vi "MIMIC RecvCommand.vi"(4 "error in":errorcluster, 7 "VISA resource name":refnum<visa-resource-name>) -> (0 "error out":errorcluster, 1 "Receive_buffer":u8[](array[numeric]), 2 "Receive Buffer_MP":u8[](array[numeric]), 3 "VISA resource name OUT":refnum<visa-resource-name>)   [LabVIEW 2014]
panel:
  out "IndexArray":u8[](array[numeric])
  out "Numeric":dbl
  out "Write Time":u32
  out "Read Time":u32
  out "return count":u32
  out "NUM_BYTES":u32
  out "Index":u32
  out "continue_flag":bool=TRUE
  out "STRT_TIME":u32
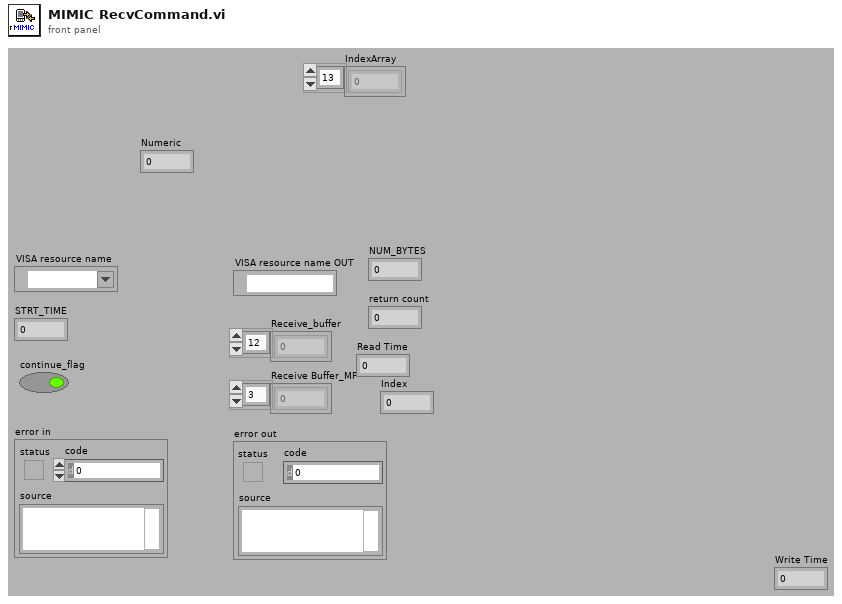
[diagram p1: front panel]
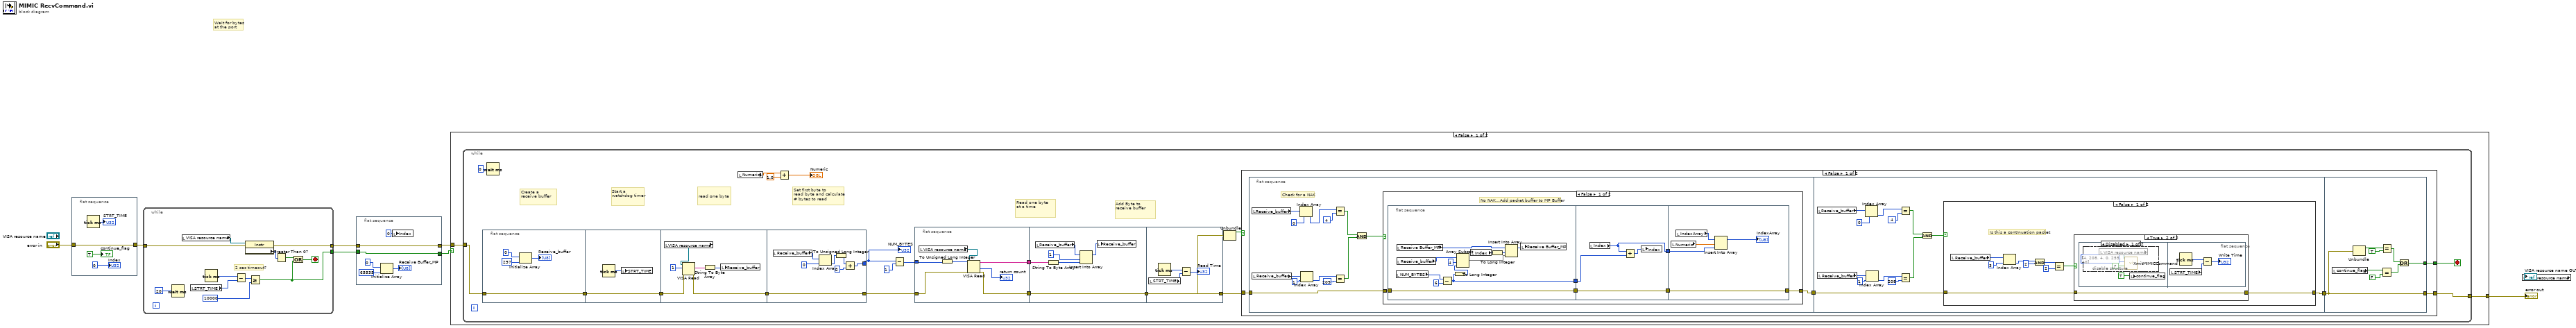
[diagram p0: block diagram]
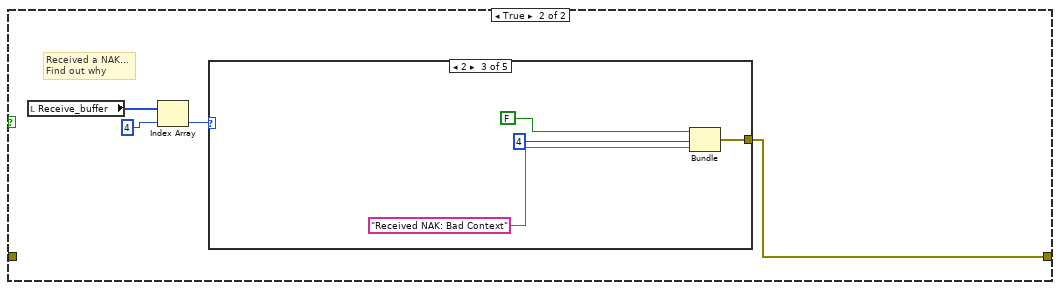
[diagram p2: hidden frame]
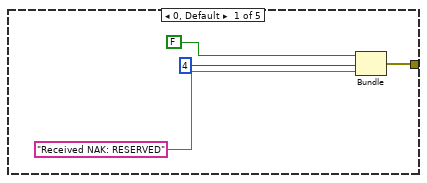
[diagram p3: hidden frame]
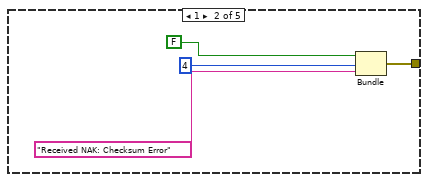
[diagram p4: hidden frame]
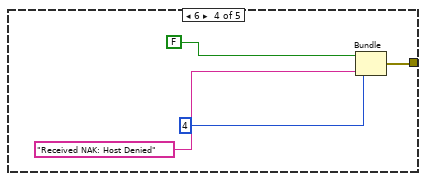
[diagram p5: hidden frame]
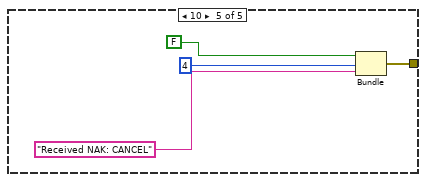
[diagram p6: hidden frame]
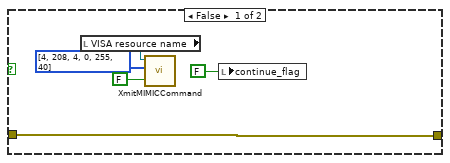
[diagram p7: hidden frame]
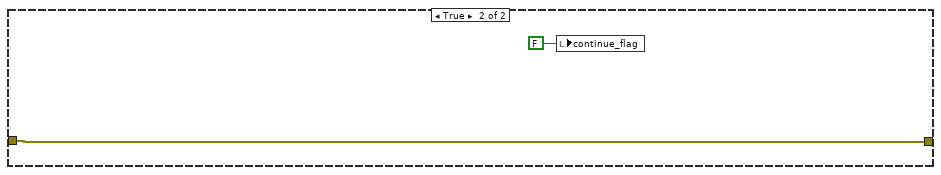
[diagram p9: hidden frame]
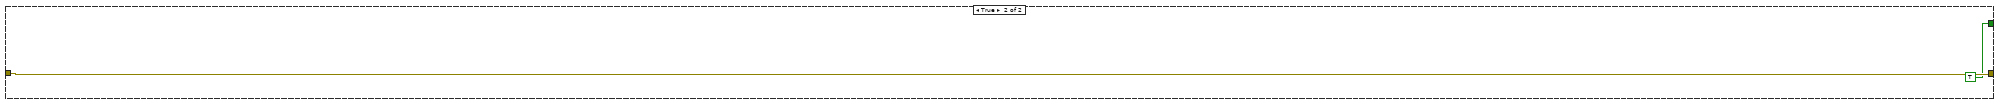
[diagram p10: hidden frame]
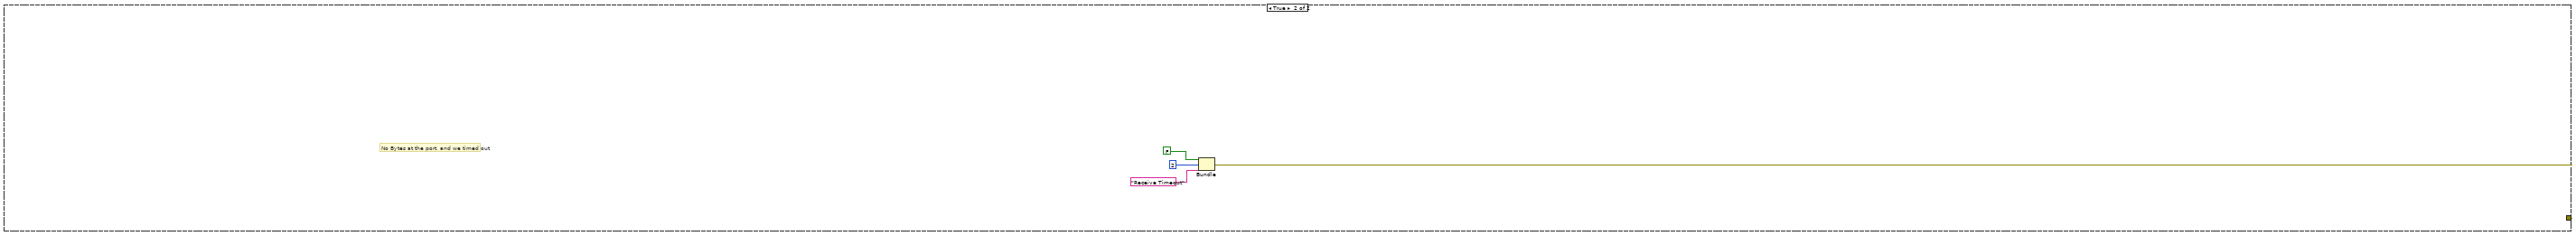
[diagram p11: hidden frame]
diagram:
  # "Wait for bytes\nat the port"
  n1 = flat-sequence {
    tunnel: "error in" -> [w11]
    tunnel: [w11] -> w6
    frame #0 {
      n2 = Tick Count (ms)() -> (millisecond timer value=→"STRT_TIME":u32)
      "continue_flag" <- TRUE
      "Index" <- u32 0
    }
  }
  n3 = while {
    tunnel: w6 -> [w21]
    tunnel: [w22] -> w4
    tunnel: [w14] -> w3
    stop <- w23 stop-if-true
    # "2 sec timeout?"
    n4 = Wait (ms)(milliseconds to wait=u32 20 ("millisecond multiple")) -> ()  [unwired: 1 out]
    n5 = local read "VISA resource name"() -> (w13:refnum<visa-resource-name>)
    n6 = local read "STRT_TIME"() -> (w15:u32)
    n7 = Tick Count (ms)() -> (millisecond timer value=w18:u32)
    n8 = Subtract(x=w18, y=w15) -> (x-y=w17:u32)
    n9 = property class="Instr"(reference=w13, error in=w21) -> (error out=w22:errorcluster, "Serial Settings:Number of Bytes at Serial Port"=w24:u32)  [unwired: 1 out]
    n10 = Greater Or Equal?(x=w17, y=u32 10000 ("milliseconds to wait")) -> (x >= y?=w14:bool)
    n11 = Greater Than 0?(x=w24) -> (x > 0?=w19:bool)
    n12 = Or(x=w19, y=w14) -> (x .or. y?=w23:bool)
  }
  n13 = flat-sequence {
    tunnel: w4 -> [w30]
    tunnel: [w30] -> w1
    tunnel: [w29] -> w2
    tunnel: w3 -> [w29]
    frame #0 {
      n14 = Initialize Array(u8 0 ("element"), 65535 ("dimension size")) -> (→"Receive Buffer_MP":u8[])
      n15 = local write "Index"(u32 0 ("Index")) -> ()
    }
  }
  n16 = case shown="False" w2 {
    tunnel: w1 -> [w32 _]
    tunnel: [w31 w204] -> w8
    frame False {
      n17 = while {
        tunnel: w32 -> [w49]
        tunnel: [w48] -> w31
        stop <- w47 stop-if-true
        # "Add Byte to \nreceive buffer"
        # "Read one byte\nat a time"
        # "Start a watchdog timer"
        # "Set first byte to \nread byte and calculate # bytes to read"
        # "read one byte"
        # "Create a\nreceive buffer"
        n18 = flat-sequence {
          tunnel: w49 -> [w188]
          tunnel: [w188] -> w51
          tunnel: w51 -> [w190]
          tunnel: [w190] -> w50
          tunnel: w50 -> [w193]
          tunnel: [w196] -> w46
          tunnel: [w203] -> w39
          tunnel: w46 -> [w203]
          tunnel: [w199] -> w38
          frame #0 {
            n19 = Initialize Array(u8 0 ("element"), 257 ("dimension size")) -> (→"Receive_buffer":u8[])
          }
          frame #1 {
            n20 = Tick Count (ms)() -> (millisecond timer value=w189:u32)
            n21 = local write "STRT_TIME"(w189) -> ()
          }
          frame #2 {
            n22 = local read "VISA resource name"() -> (w191:refnum<visa-resource-name>)
            n23 = VISA Read(VISA resource name=w191, byte count=u32 1, error in (no error)=w193) -> (read buffer=w195:string, error out=w196:errorcluster)  [unwired: 2 out]
            n24 = String To Byte Array(string=w195) -> (unsigned byte array=w192:u8[])
            n25 = local write "Receive_buffer"(w192) -> ()
          }
          frame #3 {
            n26 = local read "Receive_buffer"() -> (w200:u8[])
            n27 = Index Array(array=w200, index=0) -> (element=w198:u8)
            n28 = To Unsigned Long Integer(number=w198) -> (unsigned 32bit integer=w197:u32)
            n29 = Add(x=w197, y=u32 2) -> (x+y=w199:u32)
          }
        }
        n30 = Wait (ms)(milliseconds to wait=u32 0 ("millisecond multiple")) -> ()  [unwired: 1 out]
        n31 = local read "Numeric"() -> (w35:dbl)
        n32 = Add(x=w35, y=1.0) -> (x+y=→"Numeric":dbl)
        n33 = Subtract(x=w38, y=u32 1) -> (x-y=w40:u32)
        n34 = flat-sequence {
          tunnel: [w58] -> w43
          tunnel: [w57] -> w42
          tunnel: w40 -> [w53]
          tunnel: w39 -> [w55]
          tunnel: w43 -> [w60]
          tunnel: w42 -> [w64]
          tunnel: [w64] -> w37
          tunnel: [w68] -> w44
          tunnel: w37 -> [w68]
          frame #0 {
            n35 = local read "VISA resource name"() -> (w56:refnum<visa-resource-name>)
            n36 = To Unsigned Long Integer(number=w53) -> (unsigned 32bit integer=w54:u32)
            n37 = VISA Read(VISA resource name=w56, byte count=w54, error in (no error)=w55) -> (read buffer=w58:string, return count=→"return count":u32, error out=w57:errorcluster)  [unwired: 1 out]
          }
          frame #1 {
            n38 = local read "Receive_buffer"() -> (w62:u8[])
            n39 = String To Byte Array(string=w60) -> (unsigned byte array=w61:u8[])
            n40 = Insert Into Array(array=w62, index=1, new element=w61) -> (w63:u8[])
            n41 = local write "Receive_buffer"(w63) -> ()
          }
          frame #2 {
            n42 = local read "STRT_TIME"() -> (w65:u32)
            n43 = Tick Count (ms)() -> (millisecond timer value=w67:u32)
            n44 = Subtract(x=w67, y=w65) -> (x-y=→"Read Time":u32)
          }
        }
        n45 = Unbundle(w44) -> ("status"=w45:bool)  [unwired: 2 out]
        n46 = case shown="False" w45 {
          tunnel: w44 -> [w71 w184]
          tunnel: [w70 w184] -> w48
          tunnel: [w69 TRUE] -> w47
          frame False {
            n47 = flat-sequence {
              tunnel: w71 -> [w75]
              tunnel: [w74] -> w73
              tunnel: w73 -> [w139]
              tunnel: [w138] -> w72
              tunnel: [w175] -> w70
              tunnel: w72 -> [w175]
              tunnel: [w176] -> w69
              frame #0 {
                # "Check for a NAK"
                n48 = local read "Receive_buffer"() -> (w86:u8[])
                n49 = local read "Receive_buffer"() -> (w83:u8[])
                n50 = Index Array(array=w86, index=0) -> (element=w81:u8)
                n51 = Index Array(array=w83, index=1) -> (element=w80:u8)
                n52 = Equal?(x=w81, y=u8 4) -> (x = y?=w82:bool)
                n53 = Equal?(x=w80, y=u8 209) -> (x = y?=w79:bool)
                n54 = And(x=w82, y=w79) -> (x .and. y?=w76:bool)
                n55 = case shown="False" w76 {
                  tunnel: w75 -> [w92 _]
                  tunnel: [w90 w114] -> w74
                  frame False {
                    # "No NAK...Add packet buffer to MP Buffer"
                    n56 = flat-sequence {
                      tunnel: w92 -> [w100]
                      tunnel: [w100] -> w91
                      tunnel: [w99] -> w89
                      tunnel: w91 -> [w107]
                      tunnel: w89 -> [w106]
                      tunnel: [w107] -> w88
                      tunnel: [w105] -> w87
                      tunnel: [w113] -> w90
                      tunnel: w88 -> [w113]
                      tunnel: w87 -> [w109]
                      frame #0 {
                        n57 = local read "NUM_BYTES"() -> (w102:u32)
                        n58 = local read "Receive Buffer_MP"() -> (w96:u8[])
                        n59 = local read "Receive_buffer"() -> (w104:u8[])
                        n60 = Subtract(x=w102, y=u32 6) -> (x-y=w99:u32)
                        n61 = To Long Integer(number=w99) -> (32bit integer=w98:i32)
                        n62 = Array Subset(array=w104, index=4, length=w98) -> (w95:u8[])
                        n63 = local read "Index"() -> (w97:u32)
                        n64 = To Long Integer(number=w97) -> (32bit integer=w93:i32)
                        n65 = Insert Into Array(array=w96, index=w93, new element=w95) -> (w94:u8[])
                        n66 = local write "Receive Buffer_MP"(w94) -> ()
                      }
                      frame #1 {
                        n67 = local read "Index"() -> (w105:u32)
                        n68 = Add(x=w105, y=w106) -> (x+y=w108:u32)
                        n69 = local write "Index"(w108) -> ()
                      }
                      frame #2 {
                        n70 = local read "Numeric"() -> (w111:dbl)
                        n71 = local read "IndexArray"() -> (w112:u8[])
                        n72 = Insert Into Array(array=w112, index=w111, new element=w109) -> (→"IndexArray":u8[])
                      }
                    }
                  }
                  frame True {
                    # "Received a NAK...\nFind out why"
                    n73 = local read "Receive_buffer"() -> (w116:u8[])
                    n74 = Index Array(array=w116, index=4) -> (element=w115:u8)
                    n75 = case shown="2" w115 {
                      tunnel: [w118 w122 w126 w130 w134] -> w114
                      frame 0, Default {
                        n76 = Bundle(FALSE, 4, "Received NAK: RESERVED") -> (w118:errorcluster)  [unwired: 1 in]
                      }
                      frame 1 {
                        n77 = Bundle(FALSE, 4, "Received NAK: Checksum Error") -> (w122:errorcluster)  [unwired: 1 in]
                      }
                      frame 2 {
                        n78 = Bundle(FALSE, 4, "Received NAK: Bad Context") -> (w126:errorcluster)  [unwired: 1 in]
                      }
                      frame 6 {
                        n79 = Bundle(FALSE, 4, "Received NAK: Host Denied") -> (w130:errorcluster)  [unwired: 1 in]
                      }
                      frame 10 {
                        n80 = Bundle(FALSE, 4, "Received NAK: CANCEL") -> (w134:errorcluster)  [unwired: 1 in]
                      }
                    }
                  }
                }
              }
              frame #1 {
                n81 = local read "Receive_buffer"() -> (w144:u8[])
                n82 = local read "Receive_buffer"() -> (w143:u8[])
                n83 = Index Array(array=w144, index=0) -> (element=w142:u8)
                n84 = Index Array(array=w143, index=1) -> (element=w141:u8)
                n85 = Equal?(x=w142, y=u8 4) -> (x = y?=w148:bool)
                n86 = Equal?(x=w141, y=u8 208) -> (x = y?=w147:bool)
                n87 = And(x=w148, y=w147) -> (x .and. y?=w140:bool)
                n88 = case shown="False" w140 {
                  tunnel: w139 -> [w153 w174]
                  tunnel: [w152 w174] -> w138
                  frame False {
                    # "Is this a contInuation packet"
                    n89 = local read "Receive_buffer"() -> (w159:u8[])
                    n90 = Index Array(array=w159, index=3) -> (element=w157:u8)
                    n91 = And(x=w157, y=u8 2) -> (x .and. y?=w155:u8)
                    n92 = Equal?(x=w155, y=u8 2) -> (x = y?=w151:bool)
                    n93 = case shown="True" w151 {
                      tunnel: w153 -> [w164 w165]
                      tunnel: [w164 w165] -> w152
                      frame False {
                        n94 = local read "VISA resource name"() -> (w160:refnum<visa-resource-name>)
                        n95 = call "XmitMIMICCommand.vi"("HWHSflag"=FALSE, "Command array"=u8[] [4, 208, 4, 0, 255, 40], "VISA resource name"=w160) -> ()  [unwired: 1 in, 2 out]
                        n96 = local write "continue_flag"(FALSE ("continue_flag")) -> ()
                      }
                      frame True {
                        n97 = flat-sequence {
                          frame #0 {
                            n98 = disable-structure shown="Disabled" {
                              frame Disabled {
                                n99 = local read "VISA resource name"() -> (w167:refnum<visa-resource-name>)
                                n100 = call "XmitMIMICCommand.vi"("HWHSflag"=FALSE, "Command array"=u8[] [4, 208, 4, 0, 255, 40], "VISA resource name"=w167) -> ()  [unwired: 1 in, 2 out]
                              }
                              frame Enabled {
                              }
                            }
                            n101 = local write "continue_flag"(TRUE ("continue_flag")) -> ()
                          }
                          frame #1 {
                            n102 = local read "STRT_TIME"() -> (w170:u32)
                            n103 = Tick Count (ms)() -> (millisecond timer value=w172:u32)
                            n104 = Subtract(x=w172, y=w170) -> (x-y=→"Write Time":u32)
                          }
                        }
                      }
                    }
                  }
                  frame True {
                    n105 = local write "continue_flag"(FALSE ("continue_flag")) -> ()
                  }
                }
              }
              frame #2 {
                n106 = local read "continue_flag"() -> (w178:bool)
                n107 = Unbundle(w175) -> ("status"=w180:bool)  [unwired: 2 out]
                n108 = Equal?(x=w178, y=FALSE) -> (x = y?=w177:bool)
                n109 = Equal?(x=w180, y=TRUE) -> (x = y?=w182:bool)
                n110 = Or(x=w182, y=w177) -> (x .or. y?=w176:bool)
              }
            }
          }
          frame True {
          }
        }
        "NUM_BYTES" <- w38
      }
    }
    frame True {
      # "No Bytes at the port, and we timed out"
      n111 = Bundle(FALSE, 2, "Receive Timeout") -> (w204:errorcluster)  [unwired: 1 in]
    }
  }
  "error out" <- w8
  n112 = local read "VISA resource name"() -> (→"VISA resource name OUT":refnum<visa-resource-name>)
